vi "Self_Actuation_SubVi_AD7747_Ke2400.vi"(7 "Enable Output (T: Enable)":bool=TRUE, 8 "error in (no error)":errorcluster, 10 "Output Level (0)":dbl, 11 "VISA resource name":refnum<visa-resource-name>="GPIB0::5::INSTR") -> (0 "error out":errorcluster, 2 "Current":sgl, 3 "VISA resource name out":refnum<visa-resource-name>, 5 "Voltage Output(V()":dbl)   [LabVIEW 2012]
uses:
  All Driver/Keithley/2012_Keithley 24XX/Keithley 24XX.lvlib
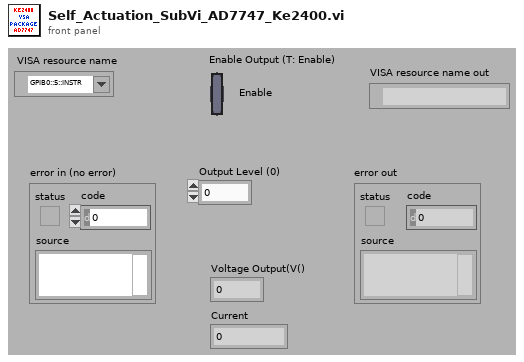
[diagram p1: front panel]
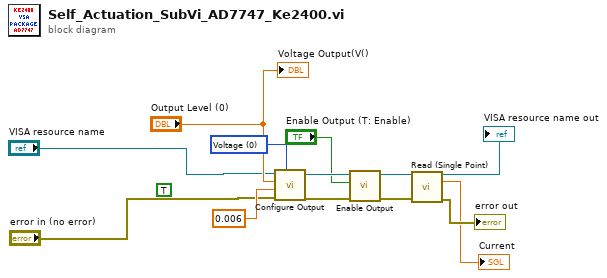
[diagram p0: block diagram]
diagram:
  w1 = u16 0 items=["Voltage", "Current"] ("Source Mode  (0: Voltage)")
  (unwired) TRUE ("Enable Auto Range (T:Enable)")
  n1 = call "Configure Output.vi"("Source Mode  (0: Voltage)"=w1, "error in (no error)"="error in (no error)", "Compliance  Level (0.1)"=0.006, "Output Level (0)"="Output Level (0)", "VISA resource name"="VISA resource name") -> ("error out"=w12:errorcluster, "VISA resource name out"=w11:refnum<visa-resource-name>)  [unwired: 5 in]
  n2 = call "Enable Output.vi"("error in (no error)"=w12, "Enable Output (T: Enable)"="Enable Output (T: Enable)", "VISA resource name"=w11) -> ("error out"=w5:errorcluster, "VISA resource name out"=w6:refnum<visa-resource-name>)  [unwired: 7 in]
  n3 = call "Read (Single Point).vi"("VISA resource name"=w6, "error in (no error)"=w5) -> ("VISA resource name out"=→"VISA resource name out":refnum<visa-resource-name>, "Current"=→"Current":sgl, "error out"=→"error out":errorcluster)  [unwired: 7 in, 4 out]
  "Voltage Output(V()" <- "Output Level (0)"
